vi "PXI-Multiplier Bank.vi"(0 "AO Channels":i32[](array[numeric]), 2 "Action":enum16{"Init", "Write", "Read"}(ring), 7 "Multipliers":dbl[](array[numeric]), 11 "error in (no error)":errorcluster) -> (4 "Channels":i32[](array[numeric]), 8 "Multipliers out":dbl[](array[numeric]), 15 "error out":errorcluster)   [LabVIEW 2020]
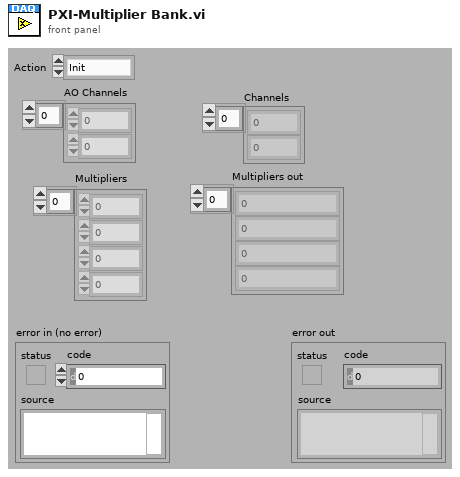
[diagram p1: front panel]
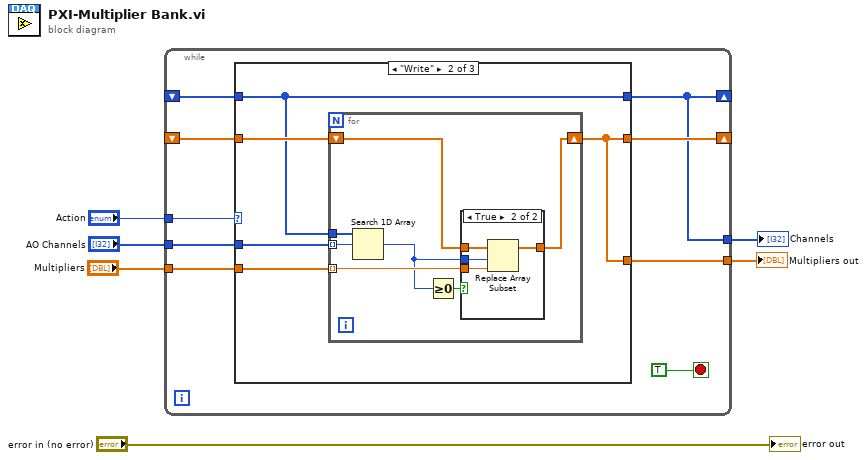
[diagram p0: block diagram]
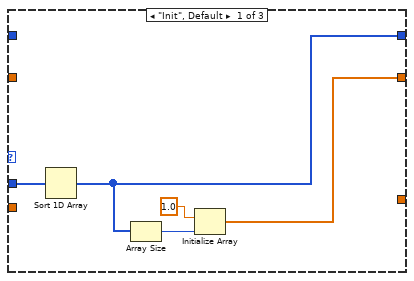
[diagram p2: hidden frame]
diagram:
  n1 = while {
    tunnel: "Action" -> [w14]
    tunnel: "AO Channels" -> [w13]
    shift-right: [w12] -> _
    shift-left: _ -> [w11]
    tunnel: "Multipliers" -> [w10]
    shift-right: [w7] -> _
    shift-left: _ -> [w9]
    tunnel: [w8] -> w2
    tunnel: [w7] -> w1
    stop <- TRUE stop-if-true
    n2 = case shown="\"Write\"" w14 {
      tunnel: w13 -> [w20 w25 _]
      tunnel: [w17 w21 w38] -> w12
      tunnel: w11 -> [_ w24 w38]
      tunnel: w10 -> [_ w23 _]
      tunnel: [w19 w22 w39] -> w7
      tunnel: w9 -> [_ w22 w39]
      tunnel: [_ w21 w38] -> w8
      frame "Init", Default {
        n3 = Sort 1D Array(array=w20) -> (sorted array=w19:i32[])
        n4 = Array Size(array=w19) -> (size(s)=w16:i32)
        n5 = Initialize Array(1.0 ("element"), w16) -> (w17:dbl[])
      }
      frame "Write" {
        n6 = for {
          tunnel: w25 -> [w28] mode=indexing
          tunnel: w23 -> [w31] mode=indexing
          tunnel: w22 -> [w29]
          shift-right: [w32] -> w21
          shift-left: w24 -> [w30]
          n7 = Search 1D Array(1D array=w29, element=w28) -> (index of element=w26:i32)  [unwired: 1 in]
          n8 = Greater Or Equal To 0?(x=w26) -> (x >= 0?=w27:bool)
          n9 = case shown="True" w27 {
            tunnel: w30 -> [w33 w37]
            tunnel: [w33 w36] -> w32
            tunnel: w26 -> [_ w35]
            tunnel: w31 -> [_ w34]
            frame False {
            }
            frame True {
              n10 = Replace Array Subset(array=w37, new element=w34, index=w35) -> (w36:dbl[])
            }
          }
        }
      }
      frame "Read" {
      }
    }
  }
  "Multipliers out" <- w2
  "Channels" <- w1
  "error out" <- "error in (no error)"
